vi "ESN_evaluateByMSE(2D array).vi"(8 "error in (no error)":errorcluster, 10 "desired Output":dbl[][](array[numeric]), 11 "Output":dbl[][](array[numeric])) -> (0 "error out":errorcluster, 3 "MSE":dbl)   [LabVIEW 2017]
uses:
  <vilib>/Analysis/NI_AALPro.lvlib
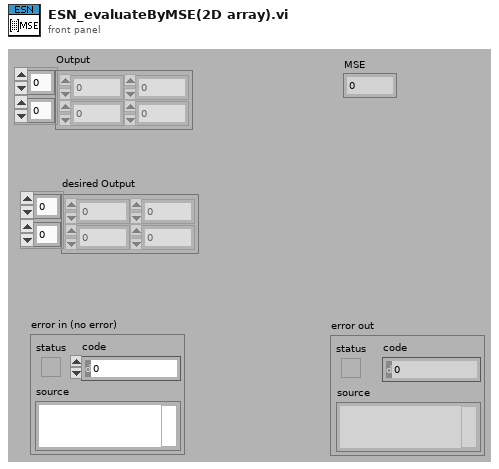
[diagram p1: front panel]
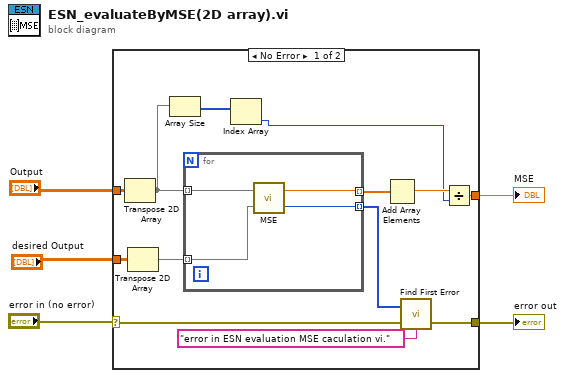
[diagram p0: block diagram]
diagram:
  n1 = case shown="No Error" "error in (no error)" {
    selector: "error in (no error)" -> [w11 w23]
    tunnel: "Output" -> [w18 _]
    tunnel: "desired Output" -> [w17 _]
    tunnel: [w13 _] -> w3
    tunnel: [w10 w23] -> w1
    frame No Error {
      n2 = Transpose 2D Array(2D array=w18) -> (transposed array=w8:dbl[][])
      n3 = Transpose 2D Array(2D array=w17) -> (transposed array=w16:dbl[][])
      n4 = Array Size(array=w8) -> (size(s)=w7:i32[])
      n5 = for {
        tunnel: w16 -> [w21] mode=indexing
        tunnel: w8 -> [w22] mode=indexing
        tunnel: [w20] -> w15 mode=indexing
        tunnel: [w19] -> w12 mode=indexing
        n6 = call <vilib>:"MSE.vi"("X Values"=w21, "Y Values"=w22) -> ("error"=w19:i32, "mse"=w20:dbl)
      }
      n7 = Index Array(array=w7) -> (element=w6:i32)  [unwired: 1 in]
      n8 = Add Array Elements(numeric array=w15) -> (sum=w14:dbl)
      n9 = call <vilib>:"Find First Error.vi"("error in (no error)"=w11, "source messages"="error in ESN evaluation MSE caculation vi.", "error codes"=w12) -> ("error out"=w10:errorcluster)  [unwired: 1 in, 1 out]
      n10 = Divide(x=w14, y=w6) -> (x/y=w13:dbl)
    }
    frame Error {
    }
  }
  "MSE" <- w3
  "error out" <- w1
